vi "Labview_code_used_in_photobleaching_and_leaching_tests.vi"() -> ()   [LabVIEW 2018]
doc: "This example demonstrates how to continuously acquire buffered voltage measurements using a DAQmx device.\n\nFor instructions on how to connect your signals to the DAQ device, refer to your device documentation."
uses:
  <vilib>/Utility/error.llb/DialogType.ctl
  <vilib>/Analysis/3filter.llb/Filter Passband Type.ctl
  <vilib>/DAQmx/read.llb/DAQmx Read (Analog Wfm 1Chan NSamp).vi
  <vilib>/Analysis/baseanly.llb/Mean (DBL).vi
  <vilib>/DAQmx/create/channels.llb/DAQmx Create Channel (AI-Voltage-Basic).vi
  <vilib>/DAQmx/configure/timing.llb/DAQmx Timing (Sample Clock).vi
  <vilib>/DAQmx/configure/trigger.llb/DAQmx Start Trigger (Digital Edge).vi
  <vilib>/DAQmx/configure/trigger.llb/DAQmx Start Trigger (Time).vi
  <vilib>/DAQmx/configure/trigger.llb/DAQmx Start Trigger (Analog Edge).vi
  <vilib>/DAQmx/miscellaneous.llb/DAQmx Fill In Error Info.vi
  <vilib>/Analysis/3filter.llb/Butterworth Filter (DBL).vi
  <vilib>/measure/maresamp.llb/Resample Waveform (single shot).vi
  <resource>/objmgr/daqmx.rc
  <vilib>/Analysis/NI_AALBase.lvlib
  <vilib>/measure/NI_MAPro.lvlib
  <vilib>/Analysis/NI_AAL_SigProc.lvlib
panel:
  in  "Confirm File Replace?":bool
  in  "File path":path=path "C:/Users/.txt"
  out "# of peaks 2":i32
  out "Resampled data 2":dbl[](graph) caption="Signal vs. Time"
  out "# of peaks":i32
  out "Waveform Graph 2":waveform(dbl)(graph) caption="Signal vs. Time"
  out "Waveform Graph":waveform(dbl)(graph) caption="Signal vs. Time"
  in  "Trigger Type":T1(tab)
  in  "Digital Start Trigger Edge":i32(ring)=10280 caption="Edge" items=["Rising"=10280, "Falling"=10171]
  in  "Digital Start Trigger Source":tag="/Dev1/PFI0" caption="Source"
  in  "Digital Pause Trigger Pause When":i32(ring)=10192 caption="Pause When" items=["High"=10192, "Low"=10214]
  in  "Digital Pause Trigger Source":tag="/Dev1/PFI0" caption="Source"
  in  "Analog Start Trigger Level":dbl caption="Level" format="%0.2f"
  in  "Analog Start Trigger Hysteresis":dbl caption="Hysteresis" format="%.2f"
  in  "Analog Start Trigger Slope":i32(ring)=10280 caption="Slope" items=["Rising"=10280, "Falling"=10171]
  in  "Analog Start Trigger Source":string="APFI0" caption="Source"
  in  "Analog Pause Trigger Source":string="APFI0" caption="Source"
  in  "Analog Pause Trigger Pause When":i32(ring)=10093 caption="Pause When" items=["Above Level"=10093, "Below Level"=10107]
  in  "Analog Pause Trigger Level":dbl caption="Level" format="%.2f"
  in  "When":timestamp
  in  "Select Time\nManually":bool
  in  "Stop":bool
  in  "Number of Samples":i32=100000
  in  "Sample Rate":dbl=200000.0
  in  "Sample Clock Source":tag="OnboardClock"
  in  "Terminal Configuration":i32(ring)=-1 items=["default"=-1, "RSE"=10083, "NRSE"=10078, "Differential"=10106, "Pseudodifferential"=12529]
  in  "Max Voltage":dbl=0.7
  in  "Min Voltage":dbl=0.5
  in  "Physical Channel":tag="myDAQ1/ai0"
  out "Actual Sample Rate":dbl=1000.0 format="%0.2f"
  # "Channel Settings"
  # "Trigger Settings"
  # "Timing Settings"
  # "To enable triggers, select a tab above, and configure the settings.\n\nNot all hardware supports all trigger types. Refer to your device documentation for more information."
  # "This trigger type is not supported in continuous sample timing. \n\nRefer to your device documentation for more information on which triggers are supported."
  # "This trigger type is not supported in continuous sample timing. \n\nRefer to your device documentation for more information on which triggers are supported."
  # "If time is not manually set, task will begin after 10 seconds"
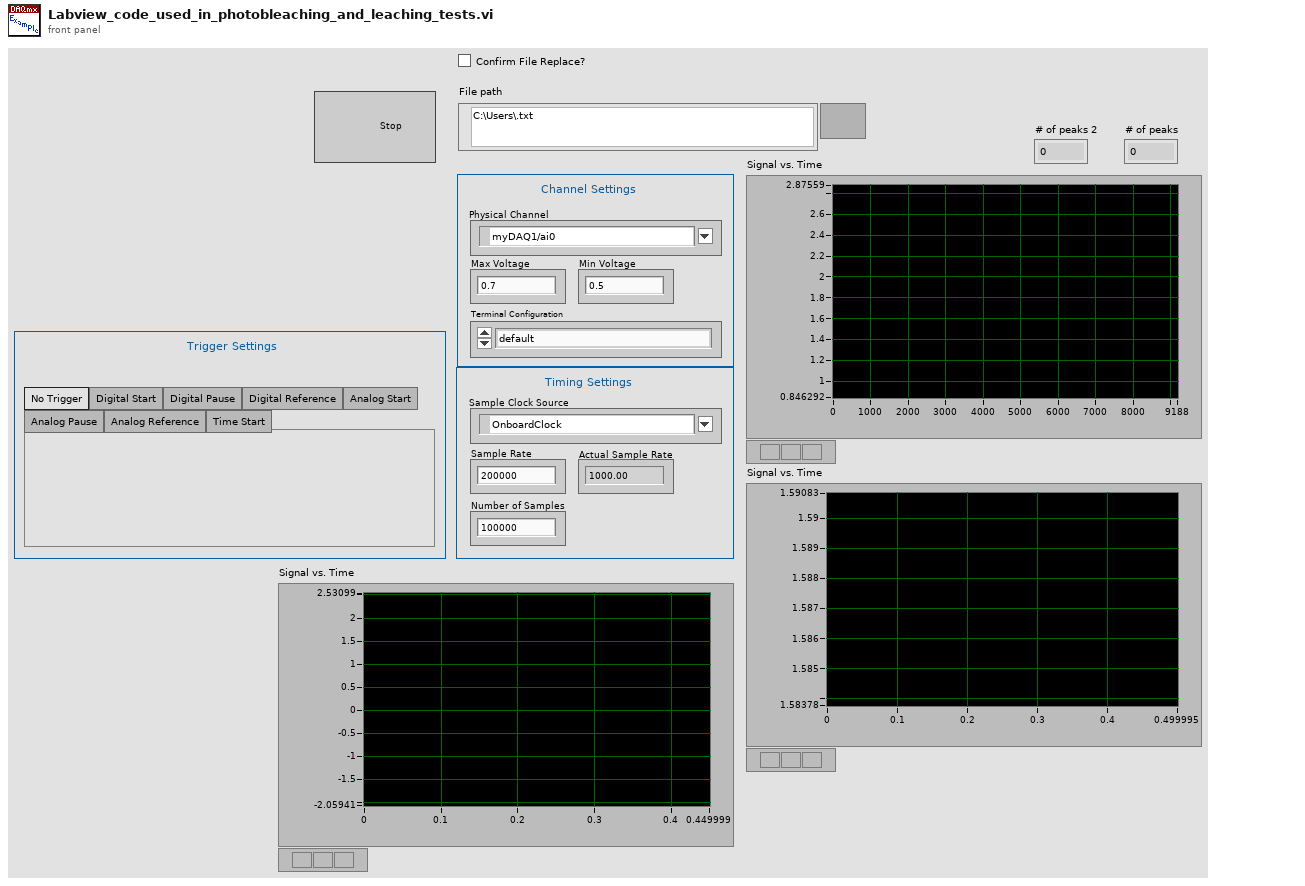
[diagram p1: front panel]
types:
  T1 = enum32{"No Trigger", "Digital Start", "Digital Pause", "Digital Reference", "Analog Start", "Analog Pause", "Analog Reference", "Time Start"}
  T2 = enum16{"open", "open or create", "create or replace", "create", "open (read only)"}
  T3 = typedef "DialogType.ctl" = u16
  T4 = cluster{"alias rejection (dB)":dbl, "normalized bandwidth":dbl}
  T5 = typedef "NI_AALBase.lvlib/Filter Passband Type.ctl" = enum32{"Lowpass", "Highpass", "Bandpass", "Bandstop"}
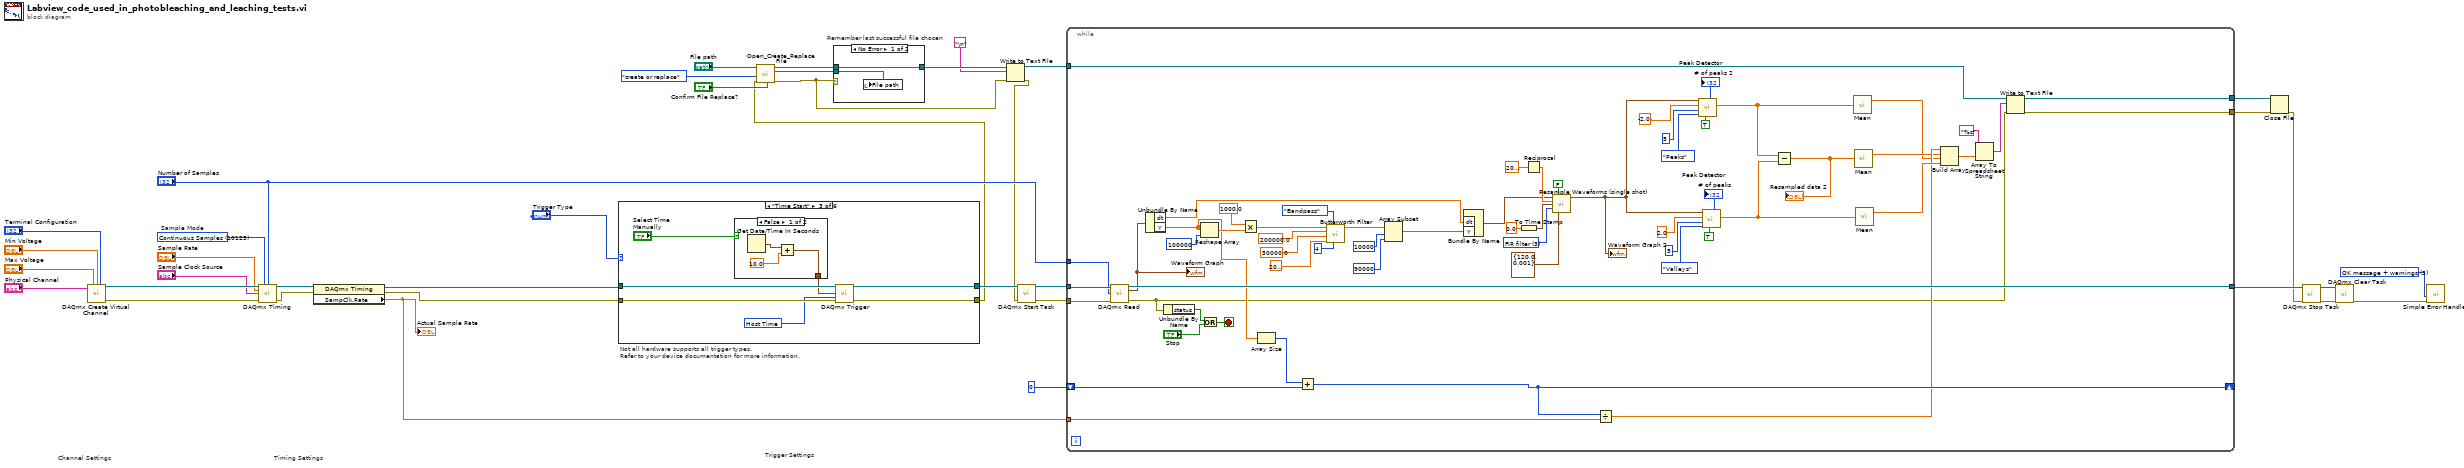
[diagram p0: block diagram]
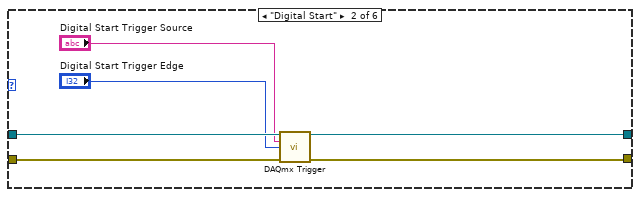
[diagram p4: hidden frame]
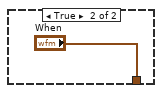
[diagram p5: hidden frame]
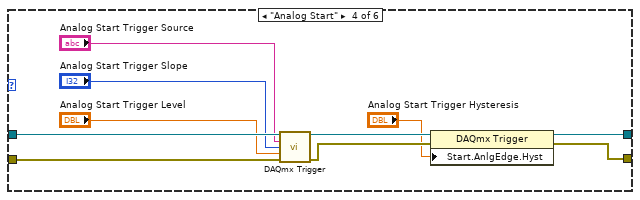
[diagram p6: hidden frame]
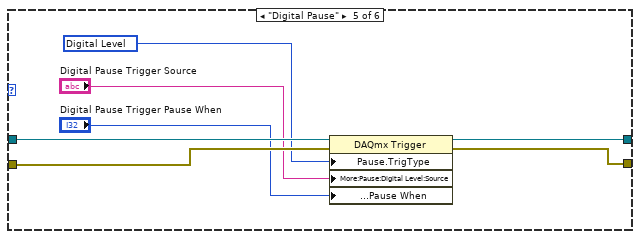
[diagram p7: hidden frame]
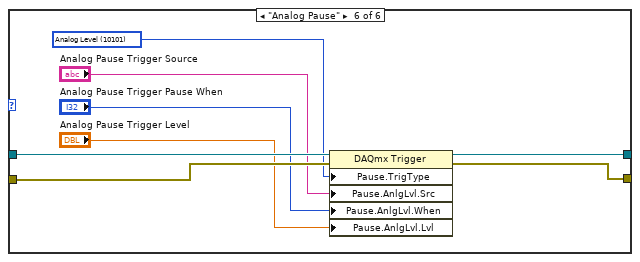
[diagram p8: hidden frame]
diagram:
  w21 = T3 3 items=["no dialog", "OK message", "continue or stop message", "OK message + warnings", "continue/stop + warnings"] ("type of dialog (OK msg:1)")
  w37 = 10123 items=["Finite Samples"=10178, "Continuous Samples"=10123, "Hardware Timed Single Point"=12522]  # Sample Mode
  # "Remember last successful file chosen"
  # "Trigger Settings"
  # "Not all hardware supports all trigger types.\nRefer to your device documentation for more information."
  # "Timing Settings"
  # "Channel Settings"
  n1 = call-poly <vilib>:"DAQmx Create Virtual Channel.vi"("maximum value"="Max Voltage", "minimum value"="Min Voltage", "input terminal configuration"="Terminal Configuration", "physical channels"="Physical Channel") -> ("task out"=w35:refnum<k21>, "error out"=w36:errorcluster)  [unwired: 10 in]
  n2 = call-poly <vilib>:"DAQmx Timing.vi"("task/channels in"=w35, "sample mode"=w37, "samples per channel"="Number of Samples", "rate"="Sample Rate", "source"="Sample Clock Source", "error in"=w36) -> ("task out"=w39:refnum<k21>, "error out"=w38:errorcluster)  [unwired: 8 in]
  n3 = property class="DAQmx Timing"(reference=w39, error in=w38) -> (reference out=w18:refnum<k21>, error out=w17:errorcluster, "SampClk.Rate"=w15:dbl)
  "Actual Sample Rate" <- w15
  n4 = case shown="\"Time Start\"" "Trigger Type" {
    tunnel: w18 -> [w41 w47 w54 w68 w75 w83]
    tunnel: w17 -> [w40 w46 w53 w67 w72 w80]
    tunnel: [w41 w45 w52 w65 w74 w82] -> w19
    tunnel: [w40 w44 w51 w64 w73 w81] -> w6
    frame "No Trigger", Default {
    }
    frame "Digital Start" {
      n5 = call-poly <vilib>:"DAQmx Trigger.vi"("task/channels in"=w47, "source"="Digital Start Trigger Source", "edge"="Digital Start Trigger Edge", "error in"=w46) -> ("task out"=w45:refnum<k21>, "error out"=w44:errorcluster)  [unwired: 10 in]
    }
    frame "Time Start" {
      w50 = 16126 items=["Host Time"=16126, "I/O Device Time"=16127] ("timescale")
      n6 = case shown="False" "Select Time\nManually" {
        tunnel: [w55 "When"] -> w48
        frame False {
          n7 = Get Date/Time In Seconds() -> (seconds since 1Jan1904=w57:timestamp)
          n8 = Add(x=w57, y=10.0) -> (x+y=w55:timestamp)
        }
        frame True {
        }
      }
      n9 = call-poly <vilib>:"DAQmx Trigger.vi"("task/channels in"=w54, "when"=w48, "timescale"=w50, "error in"=w53) -> ("task out"=w52:refnum<k21>, "error out"=w51:errorcluster)  [unwired: 10 in]
    }
    frame "Analog Start" {
      n10 = call-poly <vilib>:"DAQmx Trigger.vi"("task/channels in"=w68, "source"="Analog Start Trigger Source", "slope"="Analog Start Trigger Slope", "level"="Analog Start Trigger Level", "error in"=w67) -> ("task out"=w63:refnum<k21>, "error out"=w62:errorcluster)  [unwired: 9 in]
      n11 = property class="DAQmx Trigger"(reference=w63, error in=w62, "Start.AnlgEdge.Hyst"="Analog Start Trigger Hysteresis") -> (reference out=w65:refnum<k21>, error out=w64:errorcluster)
    }
    frame "Digital Pause" {
      w71 = 10152 items=["Analog Level"=10101, "Analog Window"=10103, "Digital Level"=10152, "Digital Pattern"=10398, "None"=10230] ("Pause.TrigType")
      n12 = property class="DAQmx Trigger"(reference=w75, error in=w72, "Pause.TrigType"=w71, "More:Pause:Digital Level:Source"="Digital Pause Trigger Source", "More:Pause:Digital Level:Pause When"="Digital Pause Trigger Pause When") -> (reference out=w74:refnum<k21>, error out=w73:errorcluster)
    }
    frame "Analog Pause" {
      w79 = 10101 items=["Analog Level"=10101, "Analog Window"=10103, "Digital Level"=10152, "Digital Pattern"=10398, "None"=10230] ("Pause.TrigType")
      n13 = property class="DAQmx Trigger"(reference=w83, error in=w80, "Pause.TrigType"=w79, "Pause.AnlgLvl.Src"="Analog Pause Trigger Source", "Pause.AnlgLvl.When"="Analog Pause Trigger Pause When", "Pause.AnlgLvl.Lvl"="Analog Pause Trigger Level") -> (reference out=w82:refnum<k21>, error out=w81:errorcluster)
    }
  }
  n14 = call <vilib>:"Open_Create_Replace File.vi"("advisory dialog? (display:T)"="Confirm File Replace?", "error in (no error)"=w6, "function (open:0)"=T2."create or replace", "file path"="File path") -> ("error out"=w5:errorcluster, "new file path"=w13:path, "refnum"=w14:refnum<file>)  [unwired: 4 in, 1 out]
  n15 = case shown="No Error" w5 {
    tunnel: w13 -> [w84 _]
    tunnel: w14 -> [w85 w86]
    tunnel: [w85 w86] -> w9
    frame No Error {
      n16 = local write "File path"(w84) -> ()
    }
    frame Error {
    }
  }
  n17 = Write to Text File(file (use dialog)=w9, text="\n", error in=w5) -> (refnum out=w7:refnum<file>, error out=w4:errorcluster)  [unwired: 1 in, 1 out]
  n18 = call <vilib>:"DAQmx Start Task.vi"("task/channels in"=w19, "error in"=w4) -> ("task out"=w34:refnum<k21>, "error out"=w33:errorcluster)  [unwired: 12 in]
  n19 = while {
    tunnel: w34 -> [w146]
    tunnel: w33 -> [w145]
    tunnel: [w144] -> w24
    tunnel: "Number of Samples" -> [w140]
    shift-right: [w124] -> _
    shift-left: 0 -> [w128]
    tunnel: w15 -> [w125]
    tunnel: w7 -> [w93]
    tunnel: [w91] -> w3
    tunnel: [w90] -> w1
    stop <- w141 stop-if-true
    w121 = u16 3 items=["coerce", "linear", "spline", "FIR filter"] ("interpolation mode")
    n20 = call-poly <vilib>:"DAQmx Read.vi"("task/channels in"=w146, "number of samples per channel"=w140, "error in"=w145) -> ("task out"=w144:refnum<k21>, "data"=w129:waveform(dbl), "error out"=w92:errorcluster)  [unwired: 10 in]
    "Waveform Graph" <- w129
    n21 = Unbundle By Name(w129) -> ("dt"=w113:dbl, "Y"=w127:dbl[])
    n22 = Unbundle By Name(w92) -> ("status"=w142:bool)
    n23 = Reshape Array(w127, 100000 ("dimension size")) -> (w130:dbl[])
    n24 = Or(x=w142, y="Stop") -> (x .or. y?=w141:bool)
    n25 = Multiply(x=1000.0, y=w130) -> (x*y=w123:dbl[])
    n26 = Array Size(array=w127) -> (size(s)=w126:i32)
    n27 = Add(x=w126, y=w128) -> (x+y=w124:i32)
    n28 = call-poly <vilib>:"Butterworth Filter.vi"("order"=4, "filter type"=Filter_Passband_Type."Bandpass", "low cutoff freq: fl"=2000.0, "high cutoff freq: fh"=30000.0, "sampling freq: fs"=200000.0, "X"=w123) -> ("Filtered X"=w122:dbl[])  [unwired: 2 in, 1 out]
    n29 = Array Subset(array=w122, index=10000, length=90000) -> (w114:dbl[])
    n30 = Bundle By Name("dt"=w113, "Y"=w114) -> (w112:waveform(dbl))  [unwired: 1 in]
    n31 = To Time Stamp(1:0.0 ("number")) -> (0:w118:timestamp)
    n32 = Reciprocal(x=2000000.0) -> (1/x=w120:dbl)
    n33 = call-poly <vilib>:"Resample Waveforms (single shot).vi"("waveform in"=w112, "open interval? (F)"=FALSE, "dt"=w120, "t0"=w118, "interpolation mode"=w121, "FIR filter specifications"=T4 {"alias rejection (dB)"=120.0, "normalized bandwidth"=0.001}) -> ("resampled waveform out"=w87:waveform(dbl))  [unwired: 6 in, 3 out]
    "Waveform Graph 2" <- w87
    n34 = Divide(x=w124, y=w125) -> (x/y=w94:dbl)
    n35 = call <vilib>:"Peak Detector.vi"("initialize (T)"=TRUE, "peaks/valleys"=enum32{"Peaks", "Valleys"}."Peaks" ("peaks/valleys 2"), "width"=5, "threshold"=-2.0, "X"=w87) -> ("Amplitudes"=w99:dbl[], "# found"=→"# of peaks 2":i32)  [unwired: 2 in, 3 out]
    n36 = call <vilib>:"Peak Detector.vi"("initialize (T)"=TRUE, "peaks/valleys"=enum32{"Peaks", "Valleys"}."Valleys" ("peaks/valleys 2"), "width"=5, "threshold"=2.0, "X"=w87) -> ("Amplitudes"=w100:dbl[], "# found"=→"# of peaks":i32)  [unwired: 2 in, 3 out]
    n37 = Subtract(x=w99, y=w100) -> (x-y=w101:dbl[])
    "Resampled data 2" <- w101
    n38 = call-poly <vilib>:"Mean.vi"("X"=w99) -> ("mean"=w88:dbl)  [unwired: 1 out]
    n39 = call-poly <vilib>:"Mean.vi"("X"=w101) -> ("mean"=w89:dbl)  [unwired: 1 out]
    n40 = call-poly <vilib>:"Mean.vi"("X"=w100) -> ("mean"=w95:dbl)  [unwired: 1 out]
    n41 = Build Array(w94, w89, w88, w95) -> (w97:dbl[])
    n42 = Array To Spreadsheet String(array=w97, 3:"%s" ("format string")) -> (spreadsheet string=w98:string)  [unwired: 1 in]
    n43 = Write to Text File(file (use dialog)=w93, text=w98, error in=w92) -> (refnum out=w90:refnum<file>, error out=w91:errorcluster)  [unwired: 1 in, 1 out]
  }
  n44 = Close File(refnum=w1, error in=w3) -> (error out=w2:errorcluster)  [unwired: 1 out]
  n45 = call <vilib>:"DAQmx Stop Task.vi"("task/channels in"=w24, "error in"=w2) -> ("task out"=w22:refnum<k21>, "error out"=w23:errorcluster)  [unwired: 12 in]
  n46 = call <vilib>:"DAQmx Clear Task.vi"("task in"=w22, "error in"=w23) -> ("error out"=w32:errorcluster)  [unwired: 13 in]
  n47 = call <vilib>:"Simple Error Handler.vi"("type of dialog (OK msg:1)"=w21, "error in (no error)"=w32) -> ()  [unwired: 3 in, 5 out]
